vi "Connect.vi"(8 "error in (no error)":errorcluster, 11 "TcpServer in":refnum<class "TcpServer.lvclass">) -> (0 "error out":errorcluster, 3 "TcpServer out":refnum<class "TcpServer.lvclass">)   [LabVIEW 2013, in "TcpServer.lvclass"]
doc: "Listens for an incoming connection. Launches a new clone of the driver to handle any incoming connections"
uses:
  TcpServer.lvclass
  TcpServer.lvclass/TcpServer.ctl
  Interface/TCP/TCP/TCP.lvclass
  TcpReader/TcpReader.lvclass
  Driver/BaseDriver/BaseDriver.lvclass
  Driver/BaseDriver/RunCaller.vi
  Driver/BaseDriver/Write Reader.vi
  Driver/BaseDriver/Write Reconnect.vi
  Driver/BaseDriver/Read Input queue.vi
  Message/BaseMessage/BaseMessage.lvclass
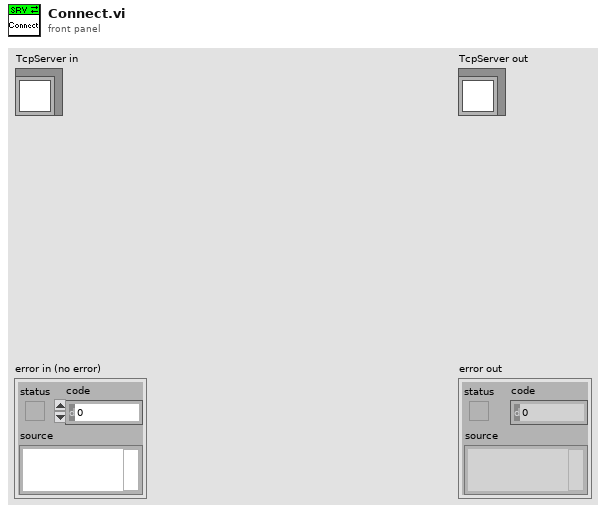
[diagram p1: front panel]
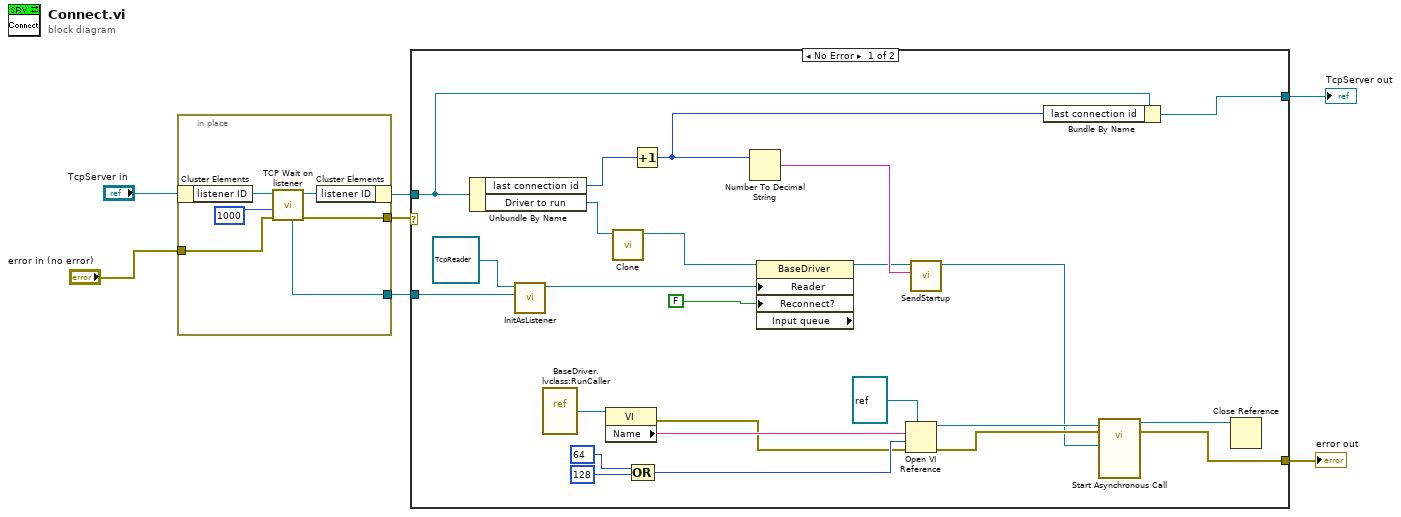
[diagram p0: block diagram]
diagram:
  n1 = in-place "In Place Element Structure" {
    in-place-border: [w10] -> w6
    in-place-border: [w9] -> w4
    in-place-border: "error in (no error)" -> [w8]
    n2 = in-place-cluster #1("TcpServer in") -> ("listener ID"=w12:refnum<class "TCP.lvclass">)
    n3 = call-dynamic "TCP Wait on listener.vi"("error in (no error)"=w8, "timeout ms (wait forever: -1)"=1000, "TCP in"=w12) -> ("error out"=w10:errorcluster, "TCP out"=w11:refnum<class "TCP.lvclass">, "connection ID"=w9:refnum<class "TCP.lvclass">)  [unwired: 4 in, 2 out]
    n4 = in-place-cluster #1("listener ID"=w11) -> (w5:refnum<class "TcpServer.lvclass">)
  }
  n5 = case shown="No Error" w6 {
    tunnel: w5 -> [w20 w38]
    tunnel: w4 -> [w36 _]
    tunnel: [w19 w38] -> w3
    tunnel: [w25 _] -> w2
    frame No Error {
      n6 = Unbundle By Name(w20) -> ("last connection id"=w23:i32, "Driver to run"=w17:refnum<class "BaseDriver.lvclass">)
      n7 = call "InitAsListener.vi"("TCP Connection"=w36, "TcpReader in"=refnum<class "TcpReader.lvclass"> refnum) -> ("TcpReader out"=w14:refnum<class "TcpReader.lvclass">)  [unwired: 8 in, 1 out]
      n8 = vi-ref "BaseDriver.lvclass:RunCaller.vi"() -> (w34:refnum<vi>)
      n9 = property on="Property Node" class="VI"(reference=w34) -> (error out=w15:errorcluster, "Name"=w33:string)  [unwired: 1 in, 1 out]
      n10 = call-dynamic "Clone.vi"("BaseDriver in"=w17) -> ("BaseDriver out"=w16:refnum<class "BaseDriver.lvclass">)  [unwired: 9 in, 1 out]
      n11 = Increment(x=w23) -> (x+1=w21:i32)
      n12 = Compound Arithmetic op=OR(64 ("options"), 128 ("options")) -> (w30:i32)
      n13 = Number To Decimal String(number=w21) -> (decimal integer string=w22:string)  [unwired: 1 in]
      n14 = property on="Property Node" class="BaseDriver" props=["Reader", "Reconnect?", "Input queue"](reference=w16, "Reader"=w14, "Reconnect?"=FALSE) -> (reference out=w18:refnum<class "BaseDriver.lvclass">)  [unwired: 1 in, 2 out]
      n15 = Open VI Reference(type specifier VI Refnum (for type only)=refnum<vi> refnum, vi path=w33, options=w30, error in (no error)=w15) -> (vi reference=w26:refnum<vi>, error out=w28:errorcluster)  [unwired: 2 in]
      n16 = call "SendStartup.vi"("Sender name"=w22, "BaseDriver in"=w18) -> ("BaseDriver out"=w24:refnum<class "BaseDriver.lvclass">)  [unwired: 8 in, 1 out]
      n17 = Bundle By Name(cluster=w20, "last connection id"=w21) -> (w19:refnum<class "TcpServer.lvclass">)
      n18 = call-by-ref "Start Asynchronous Call"(reference=w26, error in=w28, "BaseDriver in"=w24) -> (reference out=w29:refnum<vi>, error out=w25:errorcluster)  [unwired: 9 in, 2 out]
      n19 = Close Reference(reference=w29) -> ()  [unwired: 1 in, 1 out]
    }
    frame Error {
    }
  }
  "error out" <- w2
  "TcpServer out" <- w3
